vi "Get Sensor Position.vi"(8 "error in (no error)":errorcluster, 11 "Sensor in":refnum<class "Sensor.lvclass">) -> (0 "error out":errorcluster, 2 "Sensor Position":dbl[](array[numeric]), 3 "Sensor out":refnum<class "Sensor.lvclass">)   [LabVIEW 2014, in "Sensors.lvlib" / "Sensor.lvclass"]
uses:
  Sensor.lvclass
  Sensor.lvclass/Sensor.ctl
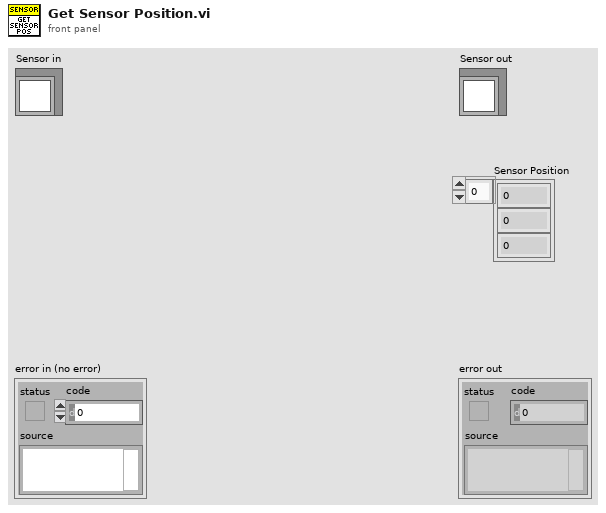
[diagram p1: front panel]
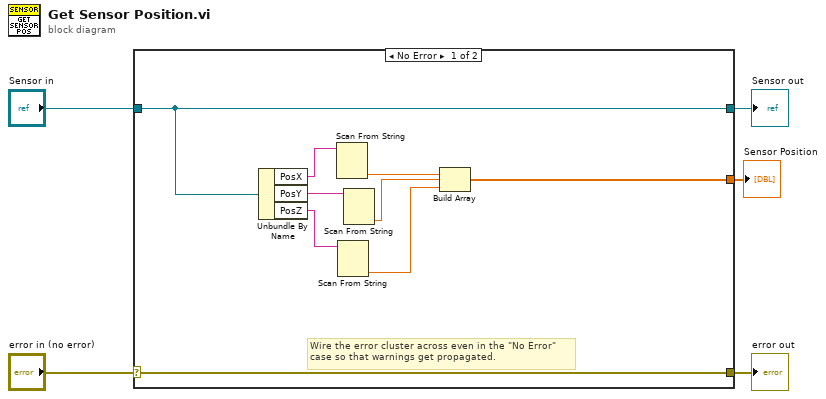
[diagram p0: block diagram]
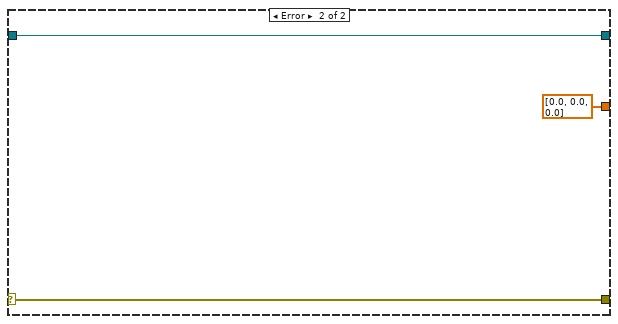
[diagram p2: hidden frame]
diagram:
  n1 = case shown="No Error" "error in (no error)" {
    selector: "error in (no error)" -> [w14 w17]
    tunnel: [w14 w17] -> w4
    tunnel: [w13 w16] -> w2
    tunnel: "Sensor in" -> [w13 w16]
    tunnel: [w6 dbl[] [0.0, 0.0, 0.0]] -> w1
    frame No Error {
      # "Wire the error cluster across even in the \"No Error\"\ncase so that warnings get propagated."
      n2 = Unbundle By Name(w13) -> ("PosX"=w12:string, "PosY"=w11:string, "PosZ"=w10:string)
      n3 = Scan From String(input string=w12) -> (output 1=w9:dbl)  [unwired: 4 in, 3 out]
      n4 = Scan From String(input string=w10) -> (output 1=w7:dbl)  [unwired: 4 in, 3 out]
      n5 = Scan From String(input string=w11) -> (output 1=w8:dbl)  [unwired: 4 in, 3 out]
      n6 = Build Array(w9, w8, w7) -> (w6:dbl[])
    }
    frame Error {
    }
  }
  "error out" <- w4
  "Sensor out" <- w2
  "Sensor Position" <- w1
